vi "getM100UPD.vi"(9 "Program":string, 10 "Product":string, 11 "Machine":string) -> (0 "UPD":i32, 1 "Second":dbl, 2 "Temp":i32, 3 "TestSec":dbl)   [LabVIEW 2012]
uses:
  <vilib>/addons/database/Connection.llb/DB Tools Open Connec (Path).vi
  <vilib>/addons/database/Connection.llb/Conn Execute.vi
  <vilib>/addons/database/Recordset.llb/Rec Fetch Integer Data (R).vi
  <vilib>/addons/database/Recordset.llb/Rec Destroy - Connection.vi
  <vilib>/addons/database/Recordset.llb/Rec Fetch Recordset Data (R).vi
  <vilib>/addons/database/_DB Variant To Data/Database Variant To Data.xnode
  <vilib>/addons/database/NI_Database_API.lvlib
panel:
  out "concatenated string 2":string
  out "x > y?":bool
  out "x .or. y?":bool
  out "substring":string
  out "concatenated string":string
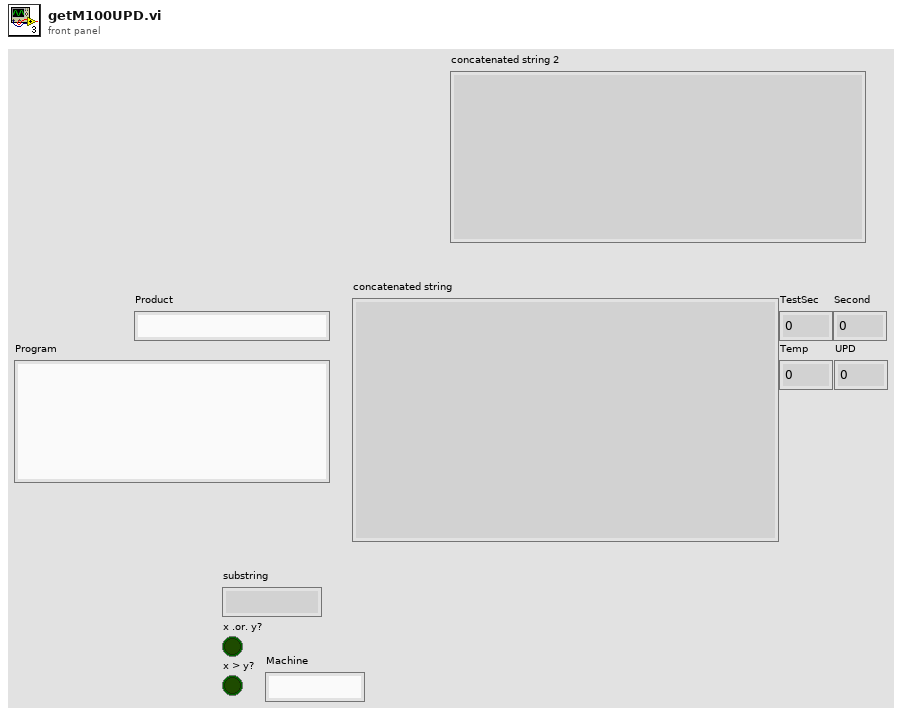
[diagram p1: front panel]
types:
  T1 = typedef "NI_Database_API.lvlib/Conn ObjectReference.ctl" = refnum<k1>
  T2 = typedef "NI_Database_API.lvlib/Rec ObjectReference.ctl" = refnum<k1>
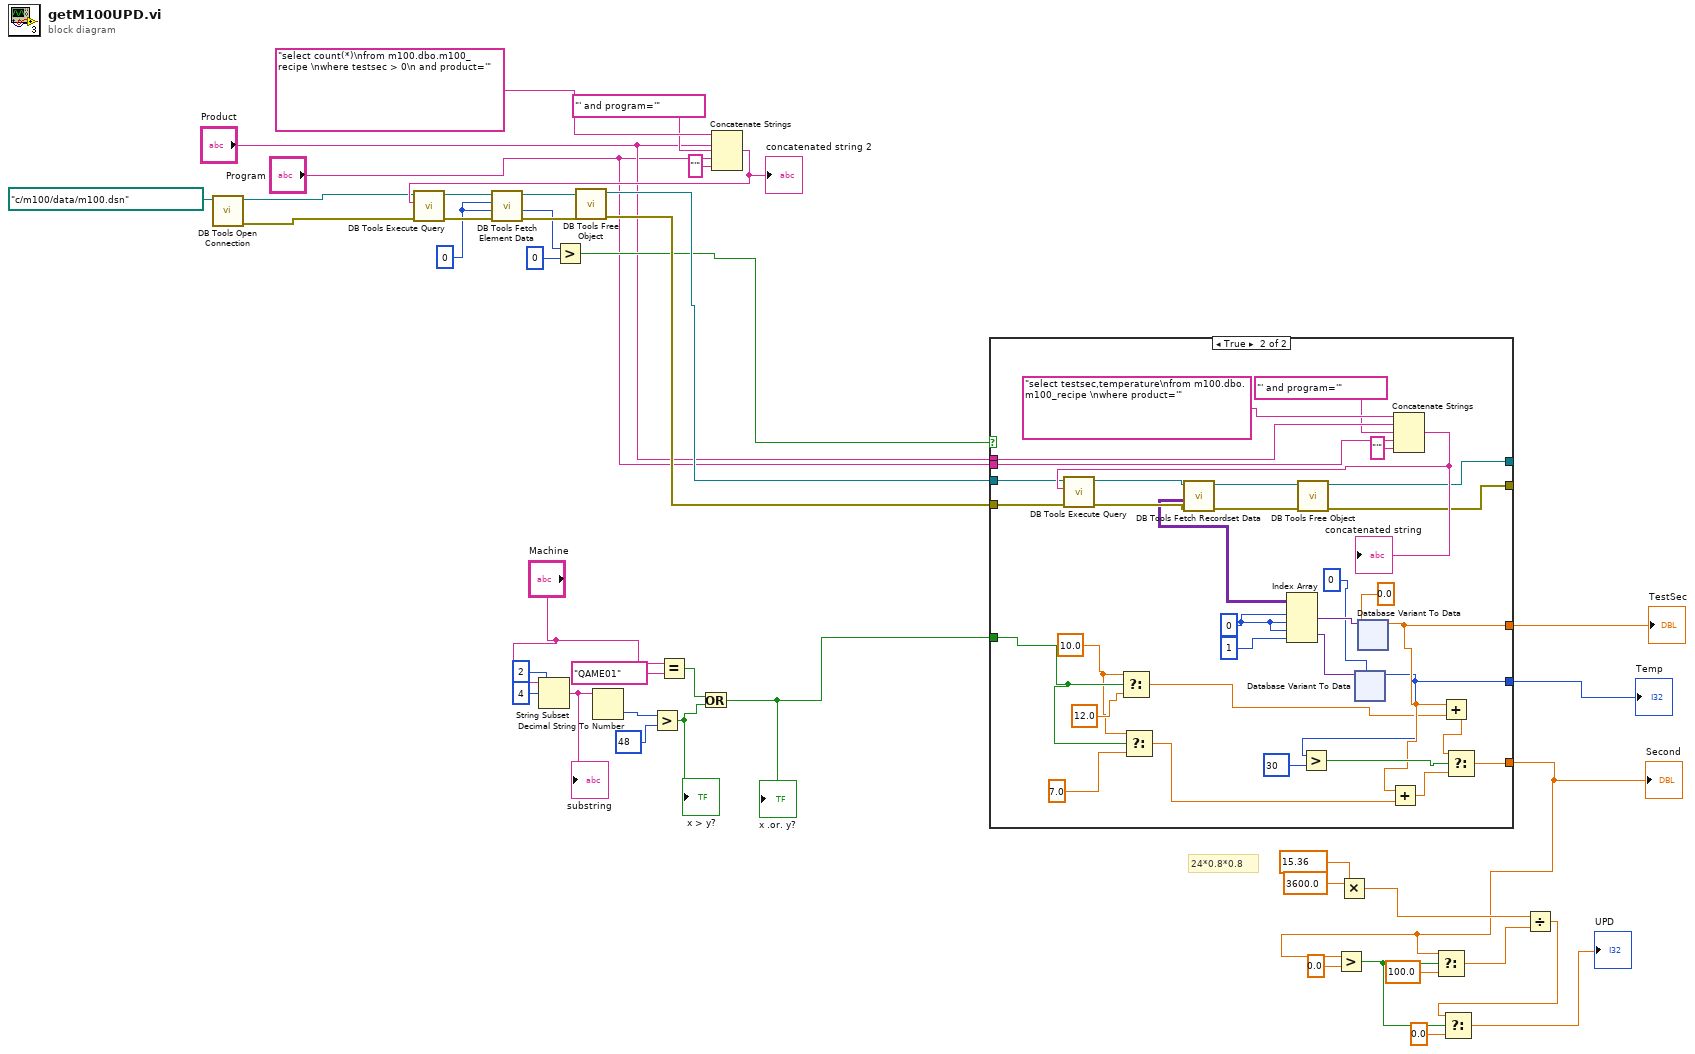
[diagram p0: block diagram]
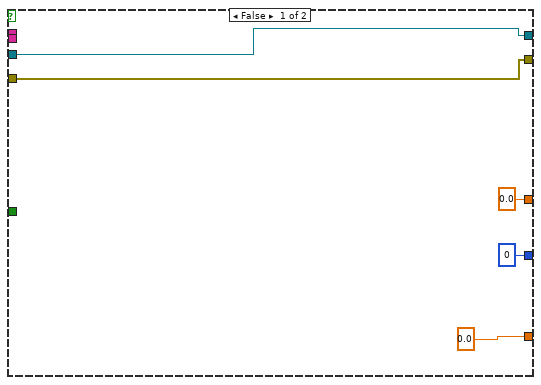
[diagram p2: hidden frame]
diagram:
  w25 = 0
  # "24*0.8*0.8"
  n1 = call-poly <vilib>:"DB Tools Open Connection.vi"("connection information"=path "c:/m100/data/m100.dsn") -> ("error out"=w21:errorcluster, "connection reference"=w22:T1)  [unwired: 7 in]
  n2 = String Subset(string="Machine", offset (0)=4, length (rest)=2 ("length (rest)")) -> (substring=w41:string)
  "substring" <- w41
  n3 = Decimal String To Number(string=w41) -> (number=w40:i32)  [unwired: 2 in, 1 out]
  n4 = Greater?(x=w40, y=48) -> (0:w36:bool)
  "x > y?" <- w36
  n5 = Equal?(x="Machine", y="QAME01") -> (x = y?=w37:bool)
  n6 = Or(x=w37, y=w36) -> (x .or. y?=w34:bool)
  "x .or. y?" <- w34
  n7 = Concatenate Strings("select count(*)\nfrom m100.dbo.m100_recipe \nwhere testsec > 0\n and product='" ("SQL query"), "Product", "' and program='" ("string"), "Program", "'" ("string")) -> (w26:string)
  "concatenated string 2" <- w26
  n8 = call-poly <vilib>:"DB Tools Execute Query.vi"("error in (no error)"=w21, "SQL query"=w26, "connection reference"=w22) -> ("error out"=w32:errorcluster, "recordset reference"=w33:T2)  [unwired: 5 in]
  n9 = call-poly <vilib>:"DB Tools Fetch Element Data.vi"("error in (no error)"=w32, "type"=w25, "column index"=w25, "recordset reference"=w33) -> ("error out"=w30:errorcluster, "data"=w24:i32, "recordset reference out"=w31:T2)  [unwired: 3 in]
  n10 = Greater?(x=w24, y=0) -> (0:w17:bool)
  n11 = call-poly <vilib>:"DB Tools Free Object.vi"("error in (no error)"=w30, "recordset reference"=w31) -> ("error out"=w18:errorcluster, "connection reference"=w19:T1)  [unwired: 8 in]
  n12 = case shown="True" w17 {
    tunnel: "Product" -> [_ w76]
    tunnel: "Program" -> [_ w74]
    tunnel: w19 -> [w47 w71]
    tunnel: w18 -> [w46 w70]
    tunnel: [w47 w69] -> _
    tunnel: [w46 w68] -> _
    tunnel: [0.0 w56] -> w3
    tunnel: [0.0 ("data") w55] -> w13
    tunnel: [0 ("data") w54] -> w12
    tunnel: w34 -> [_ w53]
    frame False {
    }
    frame True {
      w50 = 10.0 ("t")
      w65 = 0 ("disabled index (col)")
      n13 = Select(t=w50, s=w53, f=12.0 ("y")) -> (s? t:f=w51:dbl)
      n14 = Select(t=w50, s=w53, f=7.0 ("y")) -> (s? t:f=w48:dbl)
      n15 = Concatenate Strings("select testsec,temperature\nfrom m100.dbo.m100_recipe \nwhere product='" ("SQL query"), w76, "' and program='" ("string"), w74, "'" ("string")) -> (w73:string)
      "concatenated string" <- w73
      n16 = call-poly <vilib>:"DB Tools Execute Query.vi"("error in (no error)"=w70, "SQL query"=w73, "connection reference"=w71) -> ("error out"=w80:errorcluster, "recordset reference"=w81:T2)  [unwired: 5 in]
      n17 = call-poly <vilib>:"DB Tools Fetch Recordset Data.vi"("error in (no error)"=w80, "recordset reference"=w81) -> ("error out"=w78:errorcluster, "recordset data"=w67:variant[][], "recordset reference out"=w79:T2)  [unwired: 3 in]
      n18 = Index Array(array=w67, index (row) #1=w65, index (col) #1=w65, index (row) #2=w65, index (col) #2=1 ("index (col)")) -> (element #1=w64:variant, element #2=w63:variant)
      n19 = call-poly <vilib>:"DB Tools Free Object.vi"("error in (no error)"=w78, "recordset reference"=w79) -> ("error out"=w68:errorcluster, "connection reference"=w69:T1)  [unwired: 8 in]
      n20 = xnode "Database Variant To Data"("database variant"=w63, "type"=0) -> ("data"=w54:i32)  [unwired: 1 in, 1 out]
      n21 = Greater?(x=w54, y=30) -> (0:w59:bool)
      n22 = xnode "Database Variant To Data"("database variant"=w64, "type"=0.0) -> ("data"=w55:dbl)  [unwired: 1 in, 1 out]
      n23 = Add(x=w55, y=w48) -> (x+y=w57:dbl)
      n24 = Add(x=w55, y=w51) -> (x+y=w58:dbl)
      n25 = Select(t=w58, s=w59, f=w57) -> (s? t:f=w56:dbl)
    }
  }
  "TestSec" <- w13
  "Temp" <- w12
  "Second" <- w3
  n26 = Greater?(x=w3, y=0.0) -> (0:w4:bool)
  n27 = Multiply(x=3600.0, y=15.36) -> (x*y=w9:dbl)
  n28 = Select(t=w3, s=w4, f=100.0) -> (s? t:f=w2:dbl)
  n29 = Divide(x=w9, y=w2) -> (x/y=w7:dbl)
  n30 = Select(t=w7, s=w4, f=0.0) -> (s? t:f=→"UPD":dbl)
